vi "myRIO_BRig_RT__endExp_sendData.vi"(10 "input_fileName_prefix":string, 11 "input_hSession":T1) -> (0 "output_error":errorcluster, 3 "output_hSession":T1)   [LabVIEW 2014]
uses:
  <vilib>/WebDAVClient/Advanced/SessionHandle.ctl
  <vilib>/WebDAVClient/NI_WebDAV.lvlib
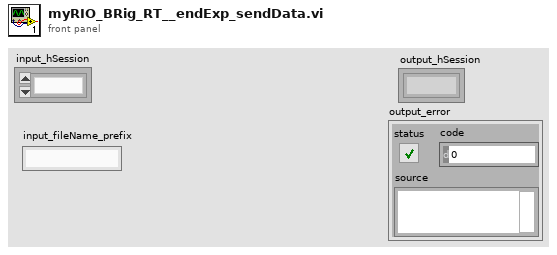
[diagram p1: front panel]
types:
  T1 = typedef "NI_WebDAV.lvlib/SessionHandle.ctl" = refnum<k1>
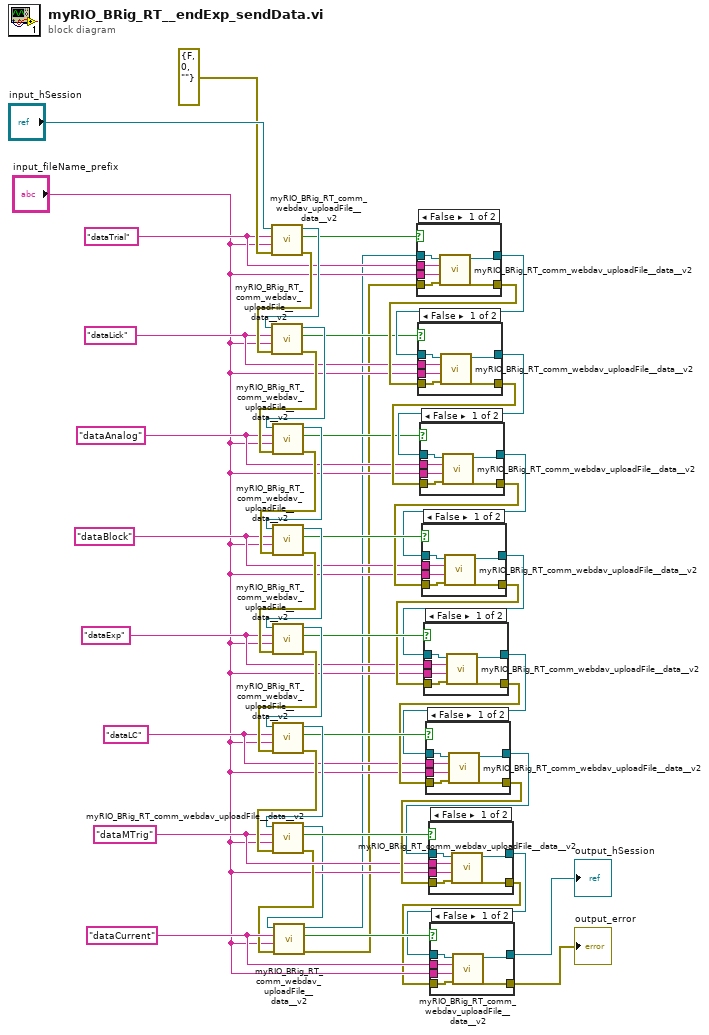
[diagram p0: block diagram]
diagram:
  w10 = "dataCurrent" ("input_filename")
  w12 = "dataMTrig" ("input_filename")
  w13 = "dataLC" ("input_filename")
  w14 = "dataExp" ("input_filename")
  w15 = "dataBlock" ("input_filename")
  w16 = "dataAnalog" ("input_filename")
  w17 = "dataLick" ("input_filename")
  w36 = "dataTrial" ("input_filename")
  n1 = call "myRIO_BRig_RT_comm_webdav_uploadFile__data__v2.vi"("input_error"=errorcluster {"status"=FALSE, "code"=0, "source"=""}, "input_fileName_prefix"="input_fileName_prefix", "input_fileName"=w36, "input_hSession"="input_hSession") -> ("output_error"=w49:errorcluster, "output_IsentFile_exp"=w37:bool, "output_hSession"=w43:T1)  [unwired: 5 in]
  n2 = call "myRIO_BRig_RT_comm_webdav_uploadFile__data__v2.vi"("input_error"=w49, "input_fileName_prefix"="input_fileName_prefix", "input_fileName"=w17, "input_hSession"=w43) -> ("output_error"=w48:errorcluster, "output_IsentFile_exp"=w31:bool, "output_hSession"=w42:T1)  [unwired: 5 in]
  n3 = call "myRIO_BRig_RT_comm_webdav_uploadFile__data__v2.vi"("input_error"=w48, "input_fileName_prefix"="input_fileName_prefix", "input_fileName"=w16, "input_hSession"=w42) -> ("output_error"=w47:errorcluster, "output_IsentFile_exp"=w30:bool, "output_hSession"=w41:T1)  [unwired: 5 in]
  n4 = call "myRIO_BRig_RT_comm_webdav_uploadFile__data__v2.vi"("input_error"=w47, "input_fileName_prefix"="input_fileName_prefix", "input_fileName"=w15, "input_hSession"=w41) -> ("output_error"=w46:errorcluster, "output_IsentFile_exp"=w29:bool, "output_hSession"=w40:T1)  [unwired: 5 in]
  n5 = call "myRIO_BRig_RT_comm_webdav_uploadFile__data__v2.vi"("input_error"=w46, "input_fileName_prefix"="input_fileName_prefix", "input_fileName"=w14, "input_hSession"=w40) -> ("output_error"=w45:errorcluster, "output_IsentFile_exp"=w26:bool, "output_hSession"=w39:T1)  [unwired: 5 in]
  n6 = call "myRIO_BRig_RT_comm_webdav_uploadFile__data__v2.vi"("input_error"=w45, "input_fileName_prefix"="input_fileName_prefix", "input_fileName"=w13, "input_hSession"=w39) -> ("output_error"=w44:errorcluster, "output_IsentFile_exp"=w23:bool, "output_hSession"=w38:T1)  [unwired: 5 in]
  n7 = call "myRIO_BRig_RT_comm_webdav_uploadFile__data__v2.vi"("input_error"=w44, "input_fileName_prefix"="input_fileName_prefix", "input_fileName"=w12, "input_hSession"=w38) -> ("output_error"=w9:errorcluster, "output_IsentFile_exp"=w20:bool, "output_hSession"=w7:T1)  [unwired: 5 in]
  n8 = call "myRIO_BRig_RT_comm_webdav_uploadFile__data__v2.vi"("input_error"=w9, "input_fileName_prefix"="input_fileName_prefix", "input_fileName"=w10, "input_hSession"=w7) -> ("output_error"=w5:errorcluster, "output_IsentFile_exp"=w11:bool, "output_hSession"=w6:T1)  [unwired: 5 in]
  n9 = case shown="False" w37 {
    tunnel: w36 -> [w57 _]
    tunnel: "input_fileName_prefix" -> [w56 _]
    tunnel: w5 -> [w55 w58]
    tunnel: w6 -> [w54 w59]
    tunnel: [w53 w59] -> w34
    tunnel: [w52 w58] -> w35
    frame False {
      n10 = call "myRIO_BRig_RT_comm_webdav_uploadFile__data__v2.vi"("input_error"=w55, "input_fileName_prefix"=w56, "input_fileName"=w57, "input_hSession"=w54) -> ("output_error"=w52:errorcluster, "output_hSession"=w53:T1)  [unwired: 5 in, 1 out]
    }
    frame True {
    }
  }
  n11 = case shown="False" w31 {
    tunnel: w17 -> [w65 _]
    tunnel: "input_fileName_prefix" -> [w64 _]
    tunnel: w35 -> [w63 w66]
    tunnel: w34 -> [w62 w67]
    tunnel: [w61 w67] -> w32
    tunnel: [w60 w66] -> w33
    frame False {
      n12 = call "myRIO_BRig_RT_comm_webdav_uploadFile__data__v2.vi"("input_error"=w63, "input_fileName_prefix"=w64, "input_fileName"=w65, "input_hSession"=w62) -> ("output_error"=w60:errorcluster, "output_hSession"=w61:T1)  [unwired: 5 in, 1 out]
    }
    frame True {
    }
  }
  n13 = case shown="False" w30 {
    tunnel: w16 -> [w73 _]
    tunnel: "input_fileName_prefix" -> [w72 _]
    tunnel: w33 -> [w71 w74]
    tunnel: w32 -> [w70 w75]
    tunnel: [w69 w75] -> w27
    tunnel: [w68 w74] -> w28
    frame False {
      n14 = call "myRIO_BRig_RT_comm_webdav_uploadFile__data__v2.vi"("input_error"=w71, "input_fileName_prefix"=w72, "input_fileName"=w73, "input_hSession"=w70) -> ("output_error"=w68:errorcluster, "output_hSession"=w69:T1)  [unwired: 5 in, 1 out]
    }
    frame True {
    }
  }
  n15 = case shown="False" w29 {
    tunnel: w15 -> [w81 _]
    tunnel: "input_fileName_prefix" -> [w80 _]
    tunnel: w28 -> [w79 w82]
    tunnel: w27 -> [w78 w83]
    tunnel: [w77 w83] -> w24
    tunnel: [w76 w82] -> w25
    frame False {
      n16 = call "myRIO_BRig_RT_comm_webdav_uploadFile__data__v2.vi"("input_error"=w79, "input_fileName_prefix"=w80, "input_fileName"=w81, "input_hSession"=w78) -> ("output_error"=w76:errorcluster, "output_hSession"=w77:T1)  [unwired: 5 in, 1 out]
    }
    frame True {
    }
  }
  n17 = case shown="False" w26 {
    tunnel: w14 -> [w89 _]
    tunnel: "input_fileName_prefix" -> [w88 _]
    tunnel: w25 -> [w87 w90]
    tunnel: w24 -> [w86 w91]
    tunnel: [w85 w91] -> w21
    tunnel: [w84 w90] -> w22
    frame False {
      n18 = call "myRIO_BRig_RT_comm_webdav_uploadFile__data__v2.vi"("input_error"=w87, "input_fileName_prefix"=w88, "input_fileName"=w89, "input_hSession"=w86) -> ("output_error"=w84:errorcluster, "output_hSession"=w85:T1)  [unwired: 5 in, 1 out]
    }
    frame True {
    }
  }
  n19 = case shown="False" w23 {
    tunnel: w13 -> [w97 _]
    tunnel: "input_fileName_prefix" -> [w96 _]
    tunnel: w22 -> [w95 w98]
    tunnel: w21 -> [w94 w99]
    tunnel: [w93 w99] -> w18
    tunnel: [w92 w98] -> w19
    frame False {
      n20 = call "myRIO_BRig_RT_comm_webdav_uploadFile__data__v2.vi"("input_error"=w95, "input_fileName_prefix"=w96, "input_fileName"=w97, "input_hSession"=w94) -> ("output_error"=w92:errorcluster, "output_hSession"=w93:T1)  [unwired: 5 in, 1 out]
    }
    frame True {
    }
  }
  n21 = case shown="False" w20 {
    tunnel: w12 -> [w105 _]
    tunnel: "input_fileName_prefix" -> [w104 _]
    tunnel: w19 -> [w103 w106]
    tunnel: w18 -> [w102 w107]
    tunnel: [w101 w107] -> w3
    tunnel: [w100 w106] -> w4
    frame False {
      n22 = call "myRIO_BRig_RT_comm_webdav_uploadFile__data__v2.vi"("input_error"=w103, "input_fileName_prefix"=w104, "input_fileName"=w105, "input_hSession"=w102) -> ("output_error"=w100:errorcluster, "output_hSession"=w101:T1)  [unwired: 5 in, 1 out]
    }
    frame True {
    }
  }
  n23 = case shown="False" w11 {
    tunnel: w10 -> [w113 _]
    tunnel: "input_fileName_prefix" -> [w112 _]
    tunnel: w4 -> [w111 w114]
    tunnel: w3 -> [w110 w115]
    tunnel: [w109 w115] -> w2
    tunnel: [w108 w114] -> w1
    frame False {
      n24 = call "myRIO_BRig_RT_comm_webdav_uploadFile__data__v2.vi"("input_error"=w111, "input_fileName_prefix"=w112, "input_fileName"=w113, "input_hSession"=w110) -> ("output_error"=w108:errorcluster, "output_hSession"=w109:T1)  [unwired: 5 in, 1 out]
    }
    frame True {
    }
  }
  "output_hSession" <- w2
  "output_error" <- w1
